vi "FuzzyEx Color Learner.vi"() -> ()   [LabVIEW 2023]
doc: "This VI uses the Fuzzy Logic VIs to train the system about your preferred color and verify the system can predict the colors you like. It also uses the Fuzzy Logic API to create rules while running and demonstrate how to save and load the new rules to a file."
uses:
  <vilib>/addons/Fuzzy Logic/TypeDefs/FL Antecedent Connective.ctl
  <vilib>/addons/Fuzzy Logic/TypeDefs/FL Consequent Implication.ctl
  <vilib>/Utility/sysdir.llb/System Directory Type.ctl
  <vilib>/addons/Fuzzy Logic/FL Fuzzy Controller (MISO).vi
  <vilib>/addons/Fuzzy Logic/NI_Fuzzy_Logic_API.lvlib
panel:
  in  "Instructions":string="Overview: This VI uses the Fuzzy Logic VIs to train the system about your preferred color and verify the system can predict the colors you like. It also uses the Fuzzy Logic API to create rules while running and demonstrate how to save and load the new rules to a file. \nInstructions:\n1. Run the VI and click Sort a color to obtain a random 'Sorted color'.\n2. Choose your opinion about this color and click Learn to train the controller.\n3. After training, sort a color again and click Guess my opinion to verify how the fuzzy system has learnt your opinions. You may be asked for more training.\n4. More consistent training will increase intelligence faster.\n5. Click Stop to stop the VI."
  in  "save":bool
  in  "load":bool
  out "Intelligence level":dbl(slide) scale=0.0..1.0
  in  "reset training":bool
  in  "stop":bool
  out "times trained":i32
  in  "sort":bool
  out "calculated opinion":string
  in  "Your opinion":T1(radio)=enum."Indifferent"
  in  "learn":bool
  in  "guess":bool
  out "Sorted color":u32(colorbox)=16777238
  # "Training section"
  # "Verify training section"
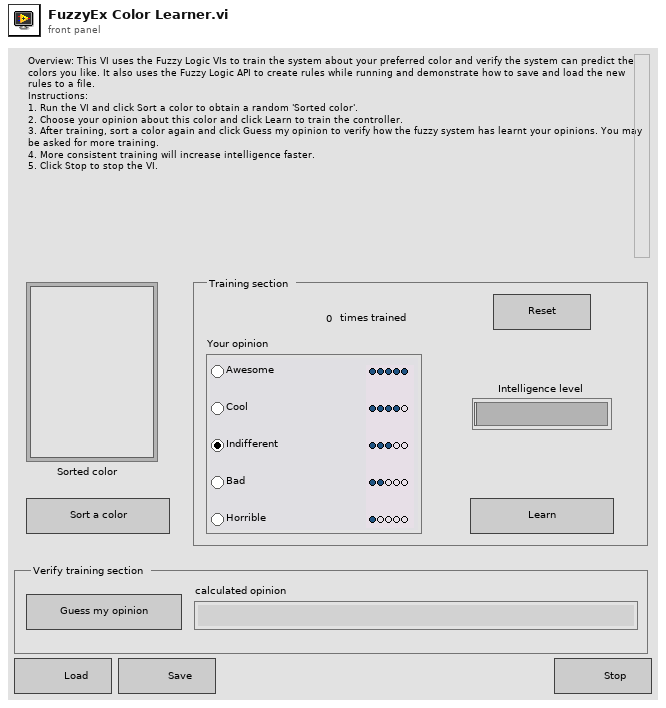
[diagram p1: front panel]
types:
  T1 = enum32{"Awesome", "Cool", "Indifferent", "Bad", "Horrible"}
  T2 = typedef "NI_Fuzzy_Logic_API.lvlib/FL System.ctl" = cluster{"input variables":T3[], "output variables":T3[], "rules":T6[], "defuzzification method":T12, "description":string, "user MF interpolating polynomials":T13[]}
  T3 = typedef "NI_Fuzzy_Logic_API.lvlib/FL Variable.ctl" = cluster{"name":string, "range":dbl[], "MFs":T4[]}
  T4 = typedef "NI_Fuzzy_Logic_API.lvlib/FL Membership Function.ctl" = cluster{"name":string, "shape":T5, "points":dbl[], "color":u32, "user-defined shape index":i32}
  T5 = typedef "NI_Fuzzy_Logic_API.lvlib/FL Membership Function Shape.ctl" = u16
  T6 = typedef "NI_Fuzzy_Logic_API.lvlib/FL Rule.ctl" = cluster{"antecedents":T7[], "antecedent connective":T9, "consequents":T10[], "consequent implication":T11, "degree of support":dbl}
  T7 = typedef "NI_Fuzzy_Logic_API.lvlib/FL Antecedent.ctl" = cluster{"Var Index":i32, "MF Index":i32, "Cond":T8}
  T8 = typedef "NI_Fuzzy_Logic_API.lvlib/FL Modifier.ctl" = u16
  T9 = typedef "NI_Fuzzy_Logic_API.lvlib/FL Antecedent Connective.ctl" = u16
  T10 = typedef "NI_Fuzzy_Logic_API.lvlib/FL Consequent.ctl" = cluster{"Var Index":i32, "MF Index":i32, "Cond":T8}
  T11 = typedef "NI_Fuzzy_Logic_API.lvlib/FL Consequent Implication.ctl" = u16
  T12 = typedef "NI_Fuzzy_Logic_API.lvlib/FL Defuzzification.ctl" = u16
  T13 = typedef "NI_Fuzzy_Logic_API.lvlib/FL Interpolating polynomials.ctl" = cluster{"X":dbl[], "Y":dbl[], "Y(x) coeff":dbl[][], "X(y) coeff":dbl[][], "Area(y) coeff":dbl[][], "coa_x(y) coeff":dbl[][]}
  T14 = typedef "System Directory Type.ctl" = i32
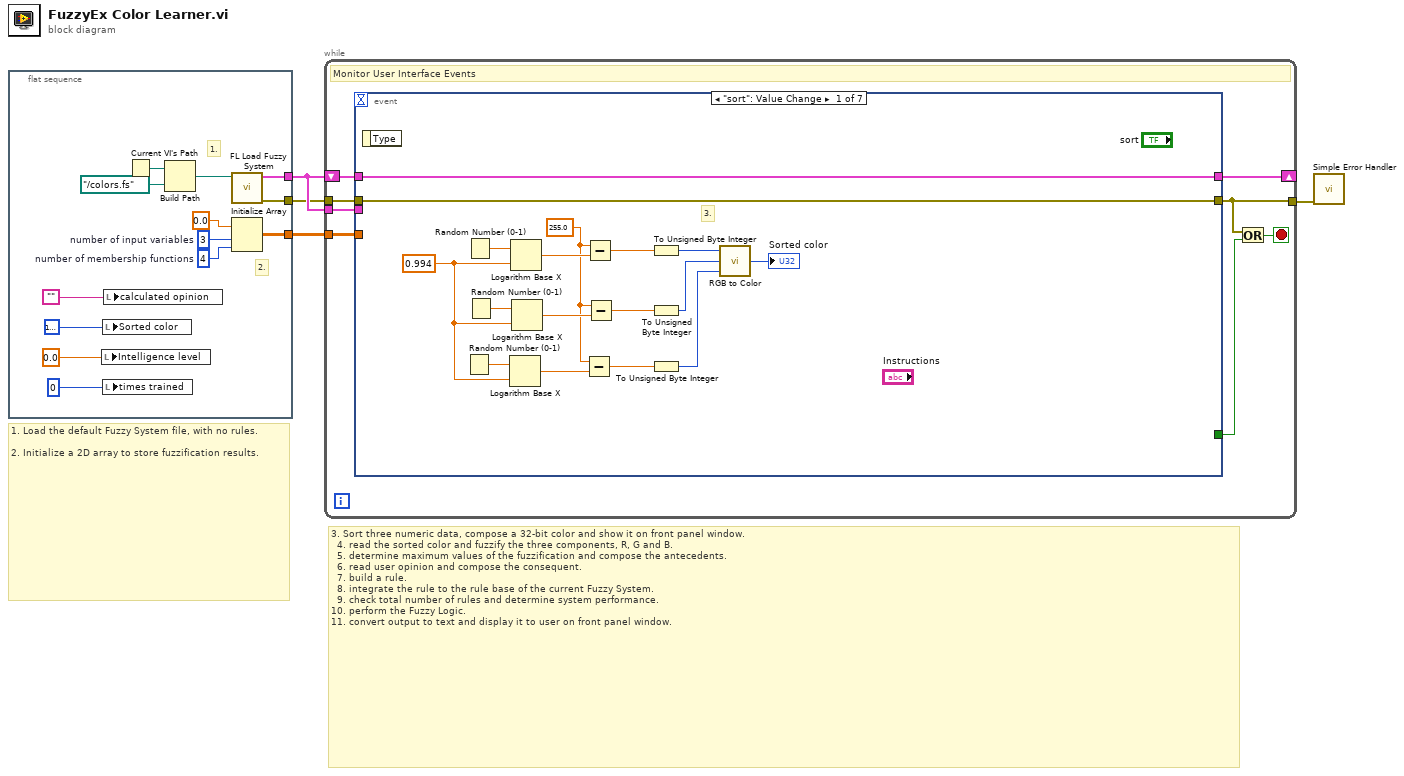
[diagram p0: block diagram]
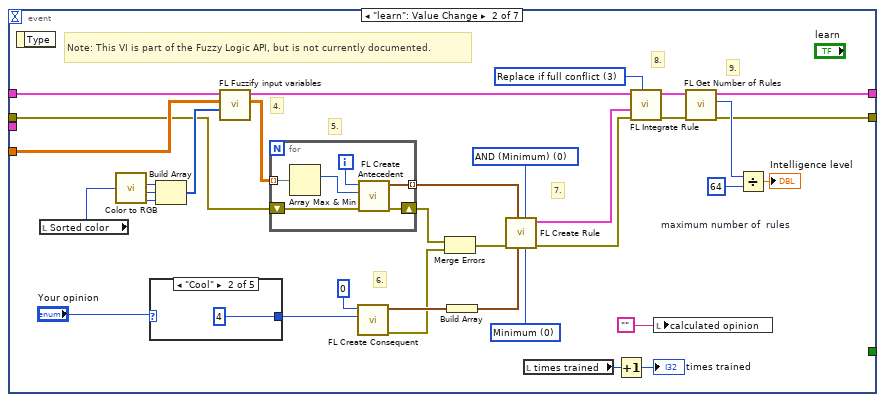
[diagram p2: hidden frame]
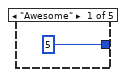
[diagram p3: hidden frame]
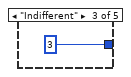
[diagram p4: hidden frame]
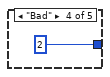
[diagram p5: hidden frame]
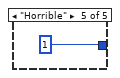
[diagram p6: hidden frame]
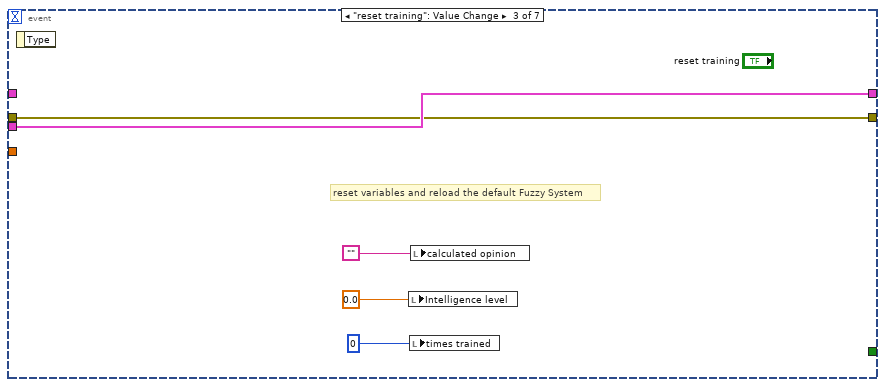
[diagram p7: hidden frame]
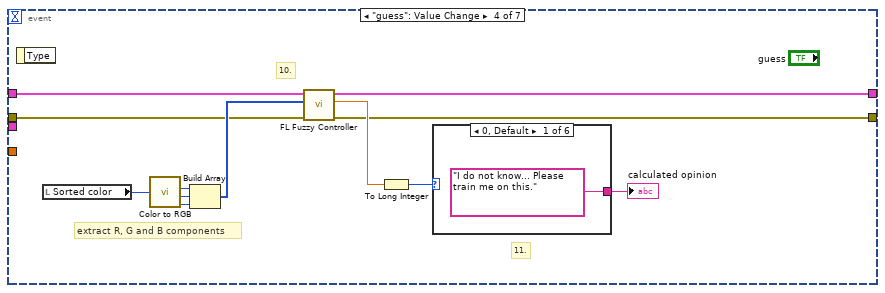
[diagram p8: hidden frame]
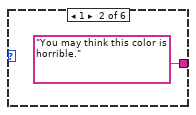
[diagram p9: hidden frame]
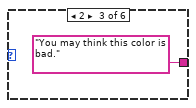
[diagram p10: hidden frame]
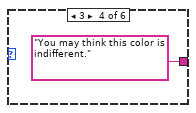
[diagram p11: hidden frame]
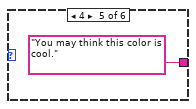
[diagram p12: hidden frame]
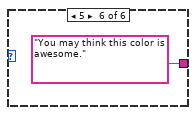
[diagram p13: hidden frame]
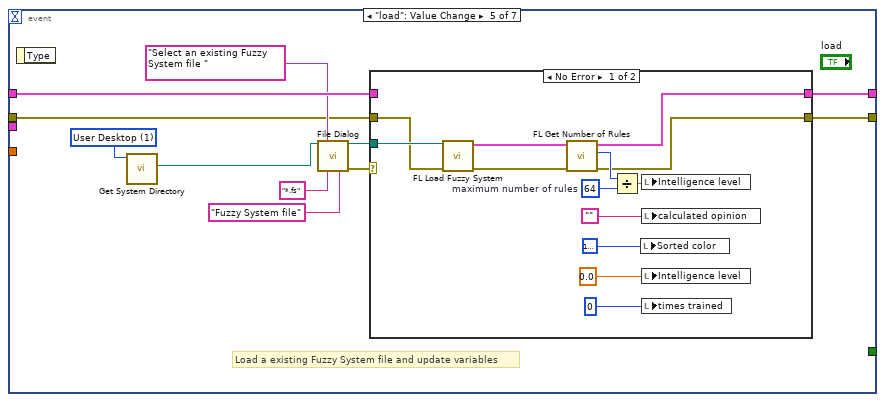
[diagram p14: hidden frame]
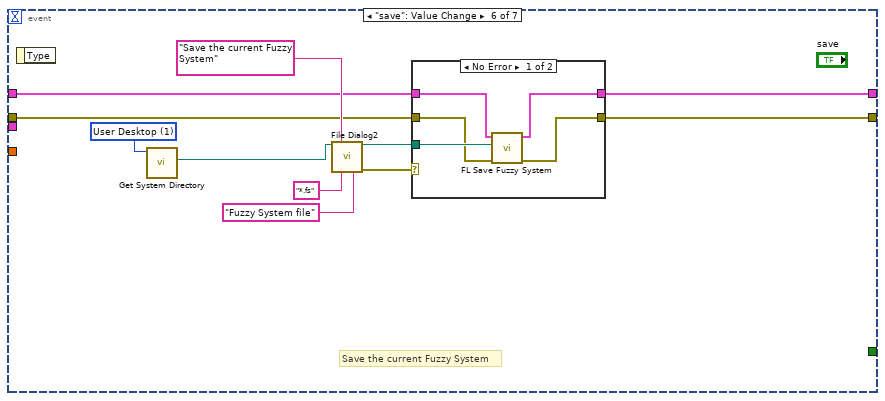
[diagram p16: hidden frame]
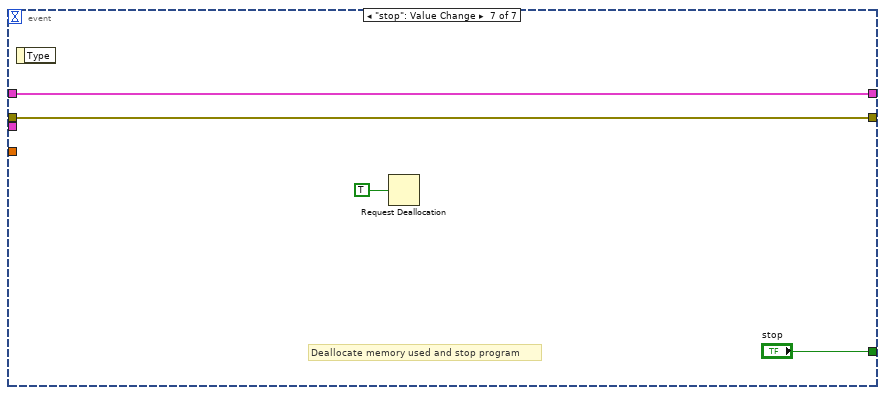
[diagram p18: hidden frame]
diagram:
  # "3. Sort three numeric data, compose a 32-bit color and show it on front panel window.\n  4. read the sorted color and fuzzify the three components, R, G and B. \n  5. determine maximum values of the fuzzification and compose the antecedents.\n  6. read user opinion and compose the consequent.\n  7. build a rule.\n  8. integrate the rule to the rule base of the current Fuzzy System.\n  9. check total number of rules and determine system performance.\n10. perform the Fuzzy Logic.\n11. convert output to text and display it to user on front panel window."
  # "1. Load the default Fuzzy System file, with no rules.\n\n2. Initialize a 2D array to store fuzzification results."
  n1 = flat-sequence {
    tunnel: [w17] -> w3
    tunnel: [w13] -> w4
    tunnel: [w5] -> w2
    frame #0 {
      w16 = 4  # number of membership functions
      w15 = 3  # number of input variables
      # "2."
      # "1."
      n2 = local write "Intelligence level"(0.0 ("times trained")) -> ()
      n3 = local write "Sorted color"(u32 16777238 ("Sorted Color")) -> ()
      n4 = local write "times trained"(0 ("times trained")) -> ()
      n5 = local write "calculated opinion"("" ("calculated opinion")) -> ()
      n6 = Current VI's Path() -> (path=w6:path)
      n7 = Build Path(base path=w6, name or relative path=path "../colors.fs") -> (appended path=w7:path)
      n8 = call <vilib>:"FL Load Fuzzy System.vi"("file path"=w7) -> ("error out"=w5:errorcluster, "fuzzy system out"=w17:T2)  [unwired: 9 in]
      n9 = Initialize Array(0.0 ("Membership"), w15, w16) -> (w13:dbl[][])
    }
  }
  n10 = while {
    tunnel: w4 -> [w24]
    shift-right: [w23] -> _
    shift-left: w3 -> [w25]
    tunnel: w3 -> [w22]
    tunnel: w2 -> [w21]
    tunnel: [w18] -> w1
    stop <- w20 stop-if-true
    # "Monitor User Interface Events"
    n11 = event shown="[0] \"sort\": Value Change" {
      selector: _ -> [_ _ _ _ _ _ _]
      dyn-events: _ -> [_ _ _ _ _ _ _]
      timeout: _ -> [_ _ _ _ _ _ _]
      tunnel: [_ _ _ _ _ _ "stop"] -> w19
      tunnel: w25 -> [w39 w76 _ w104 w119 w142 w157]
      tunnel: w24 -> [_ w70 _ _ _ _ _]
      tunnel: [w39 w55 w92 w95 w118 w139 w157] -> w23
      tunnel: w22 -> [_ _ w92 _ _ _ _]
      tunnel: w21 -> [w26 w43 w88 w94 w112 w138 w155]
      tunnel: [w26 w44 w88 w93 w111 w137 w155] -> w18
      event "sort": Value Change {
        w30 = 0.994 ("x")
        w27 = 255.0 ("y")
        # "3."
        n12 = event-data() -> ()  [unwired: 1 in, 1 out]
        n13 = Random Number (0-1)() -> (number: 0 to 1=w33:dbl)
        n14 = Random Number (0-1)() -> (number: 0 to 1=w38:dbl)
        n15 = Random Number (0-1)() -> (number: 0 to 1=w34:dbl)
        n16 = Logarithm Base X(1:w30, 2:w33) -> (0:w32:dbl)
        n17 = Logarithm Base X(1:w30, 2:w38) -> (0:w37:dbl)
        n18 = Logarithm Base X(1:w30, 2:w34) -> (0:w35:dbl)
        n19 = Subtract(x=w27, y=w32) -> (x-y=w31:dbl)
        n20 = Subtract(x=w27, y=w37) -> (x-y=w36:dbl)
        n21 = Subtract(x=w27, y=w35) -> (x-y=w29:dbl)
        n22 = To Unsigned Byte Integer(number=w36) -> (unsigned 8bit integer=w40:u8)
        n23 = To Unsigned Byte Integer(number=w29) -> (unsigned 8bit integer=w41:u8)
        n24 = To Unsigned Byte Integer(number=w31) -> (unsigned 8bit integer=w42:u8)
        n25 = call <vilib>:"RGB to Color.vi"("B"=w42, "G"=w41, "R"=w40) -> ("Color"=→"Sorted color":u32)
      }
      event "learn": Value Change {
        w53 = 64  # maximum number of  rules
        w54 = u16 3 items=["Check rule only", "Add if no conflicts", "Add if partial conflicts", "Replace if full conflict"] ("integration option")
        w62 = T11 0 items=["Minimum", "Product"] ("consequent implication")
        w63 = T9 0 items=["AND (Minimum)", "AND (Product)", "OR (Maximum)", "OR (Probabilistic)"] ("antecedent connective")
        # "Note: This VI is part of the Fuzzy Logic API, but is not currently documented."
        # "9."
        # "8."
        # "7."
        # "6."
        # "5."
        # "4."
        n26 = event-data() -> ()  [unwired: 1 in, 1 out]
        n27 = local read "Sorted color"() -> (w75:u32)
        n28 = call <vilib>:"Color to RGB.vi"("Color"=w75) -> ("R"=w74:u8, "G"=w73:u8, "B"=w72:u8)  [unwired: 1 out]
        n29 = case shown="\"Cool\"" "Your opinion" {
          tunnel: [5 4 3 2 1] -> w67
          frame "Awesome" {
          }
          frame "Cool" {
          }
          frame "Indifferent" {
          }
          frame "Bad" {
          }
          frame "Horrible" {
          }
        }
        n30 = Build Array(w74, w73, w72) -> (w71:u8[])
        n31 = call <vilib>:"FL Fuzzify input variables.vi"("Input Variables"=w71, "input membership factors (u)"=w70, "fuzzy system in"=w76) -> ("membership factors (u)"=w69:dbl[][], "fuzzy system out"=w61:T2)  [unwired: 1 in, 6 out]
        n32 = for {
          tunnel: w69 -> [w87] mode=indexing
          tunnel: [w84] -> w65 mode=indexing
          shift-right: [w83] -> w49
          shift-left: w43 -> [w82]
          i -> [w86]
          n33 = Array Max & Min(array=w87) -> (max index (indices)=w85:i32)  [unwired: 3 out]
          n34 = call <vilib>:"FL Create Antecedent.vi"("error in (no error)"=w82, "membership function index"=w85, "variable index"=w86) -> ("error out"=w83:errorcluster, "antecedent"=w84:T7)  [unwired: 7 in]
        }
        n35 = call <vilib>:"FL Create Consequent.vi"("membership function index"=w67, "variable index"=0) -> ("error out"=w47:errorcluster, "consequent"=w66:T10)  [unwired: 8 in]
        n36 = Merge Errors(w49, w47) -> (w48:errorcluster)
        n37 = Build Array(w66) -> (w64:T10[])
        n38 = call <vilib>:"FL Create Rule.vi"("consequent implication"=w62, "antecedent connective"=w63, "consequents"=w64, "antecedents"=w65, "error in (no error)"=w48) -> ("error out"=w46:errorcluster, "rule"=w60:T6)  [unwired: 5 in]
        n39 = local read "times trained"() -> (w59:i32)
        n40 = Increment(x=w59) -> (x+1=→"times trained":i32)
        n41 = call <vilib>:"FL Integrate Rule.vi"("integration option"=w54, "error in (no error)"=w46, "new rule"=w60, "fuzzy system in"=w61) -> ("error out"=w45:errorcluster, "fuzzy system out"=w56:T2)  [unwired: 4 in, 2 out]
        n42 = local write "calculated opinion"("" ("calculated opinion")) -> ()
        n43 = call <vilib>:"FL Get Number of Rules.vi"("error in (no error)"=w45, "fuzzy system in"=w56) -> ("error out"=w44:errorcluster, "number of rules"=w52:i32, "fuzzy system out"=w55:T2)  [unwired: 7 in]
        n44 = Divide(x=w52, y=w53) -> (x/y=→"Intelligence level":dbl)
      }
      event "reset training": Value Change {
        # "reset variables and reload the default Fuzzy System"
        n45 = event-data() -> ()  [unwired: 1 in, 1 out]
        n46 = local write "Intelligence level"(0.0 ("times trained")) -> ()
        n47 = local write "times trained"(0 ("times trained")) -> ()
        n48 = local write "calculated opinion"("" ("calculated opinion")) -> ()
      }
      event "guess": Value Change {
        # "extract R, G and B components"
        # "11."
        # "10."
        n49 = event-data() -> ()  [unwired: 1 in, 1 out]
        n50 = local read "Sorted color"() -> (w103:u32)
        n51 = call <vilib>:"Color to RGB.vi"("Color"=w103) -> ("R"=w102:u8, "G"=w101:u8, "B"=w100:u8)  [unwired: 1 out]
        n52 = Build Array(w102, w101, w100) -> (w99:u8[])
        n53 = call-poly <vilib>:"FL Fuzzy Controller.vi"("error in (no error)"=w94, "input values"=w99, "fuzzy system in"=w104) -> ("error out"=w93:errorcluster, "output value"=w97:dbl, "fuzzy system out"=w95:T2)  [unwired: 4 in, 2 out]
        n54 = To Long Integer(number=w97) -> (32bit integer=w98:i32)
        n55 = case shown="0, Default" w98 {
          tunnel: ["I do not know... Please train me on this." ("L10n_calculated opinion 0") "You may think this color is horrible." ("L10n_calculated opinion 1") "You may think this color is bad." ("L10n_calculated opinion 2") "You may think this color is indifferent." ("L10n_calculated opinion 3") "You may think this color is cool." ("L10n_calculated opinion 4") "You may think this color is awesome." ("L10n_calculated opinion 5")] -> w96
          frame 0, Default {
          }
          frame 1 {
          }
          frame 2 {
          }
          frame 3 {
          }
          frame 4 {
          }
          frame 5 {
          }
        }
        "calculated opinion" <- w96
      }
      event "load": Value Change {
        w114 = T14 1 items=["User Home", "User Desktop", "User Documents", "User Application Data", "User Preferences", "User Temporary", "Public Documents", "Public Application Data", "Public Preferences", "System Core Libraries", "System Installed Libraries", "Application Files", "Boot Volume Root"] ("system directory type")
        # "Load a existing Fuzzy System file and update variables"
        n56 = event-data() -> ()  [unwired: 1 in, 1 out]
        n57 = call <vilib>:"Get System Directory.vi"("system directory type"=w114) -> ("system directory"=w113:path)  [unwired: 10 in]
        n58 = call "File Dialog"("start path"=w113, "prompt"="Select an existing Fuzzy System file " ("L10n_select_prompt"), "pattern (all files)"="*.fs", "pattern label"="Fuzzy System file") -> ("selected path"=w116:path, "error out"=w115:errorcluster)  [unwired: 8 in, 2 out]
        n59 = case shown="No Error" w115 {
          tunnel: w119 -> [_ w136]
          tunnel: [w125 w136] -> w118
          tunnel: w116 -> [w134 _]
          tunnel: w112 -> [w123 w135]
          tunnel: [w122 w135] -> w111
          frame No Error {
            w128 = 64  # maximum number of rules
            n60 = call <vilib>:"FL Load Fuzzy System.vi"("error in (no error)"=w123, "file path"=w134) -> ("error out"=w124:errorcluster, "fuzzy system out"=w126:T2)  [unwired: 8 in]
            n61 = call <vilib>:"FL Get Number of Rules.vi"("error in (no error)"=w124, "fuzzy system in"=w126) -> ("error out"=w122:errorcluster, "number of rules"=w127:i32, "fuzzy system out"=w125:T2)  [unwired: 7 in]
            n62 = Divide(x=w127, y=w128) -> (x/y=w129:dbl)
            n63 = local write "Sorted color"(u32 16777238 ("Sorted Color")) -> ()
            n64 = local write "Intelligence level"(w129) -> ()
            n65 = local write "calculated opinion"("" ("calculated opinion")) -> ()
            n66 = local write "Intelligence level"(0.0 ("times trained")) -> ()
            n67 = local write "times trained"(0 ("times trained")) -> ()
          }
          frame Error {
          }
        }
      }
      event "save": Value Change {
        w141 = T14 1 items=["User Home", "User Desktop", "User Documents", "User Application Data", "User Preferences", "User Temporary", "Public Documents", "Public Application Data", "Public Preferences", "System Core Libraries", "System Installed Libraries", "Application Files", "Boot Volume Root"] ("system directory type")
        # "Save the current Fuzzy System"
        n68 = event-data() -> ()  [unwired: 1 in, 1 out]
        n69 = call <vilib>:"Get System Directory.vi"("system directory type"=w141) -> ("system directory"=w140:path)  [unwired: 10 in]
        n70 = call "File Dialog2"("start path"=w140, "prompt"="Save the current Fuzzy System" ("L10n_save_prompt"), "pattern (all files)"="*.fs", "pattern label"="Fuzzy System file") -> ("selected path"=w144:path, "error out"=w143:errorcluster)  [unwired: 8 in, 2 out]
        n71 = case shown="No Error" w143 {
          tunnel: w142 -> [w152 w154]
          tunnel: [w150 w154] -> w139
          tunnel: w144 -> [w151 _]
          tunnel: w138 -> [w149 w153]
          tunnel: [w148 w153] -> w137
          frame No Error {
            n72 = call <vilib>:"FL Save Fuzzy System.vi"("error in (no error)"=w149, "file path"=w151, "fuzzy system in"=w152) -> ("error out"=w148:errorcluster, "fuzzy system out"=w150:T2)  [unwired: 7 in]
          }
          frame Error {
          }
        }
      }
      event "stop": Value Change {
        # "Deallocate memory used and stop program"
        n73 = event-data() -> ()  [unwired: 1 in, 1 out]
        n74 = Request Deallocation(TRUE ("flag")) -> ()
      }
    }
    n75 = Or(x=w18, y=w19) -> (x .or. y?=w20:bool)
  }
  n76 = call <vilib>:"Simple Error Handler.vi"("error in (no error)"=w1) -> ()  [unwired: 4 in, 5 out]
